vi "Read Best Solution.vi"(8 "error in (no error)":errorcluster, 11 "SA in":refnum<class "SA.lvclass">) -> (0 "error out":errorcluster, 2 "Solution":T1, 3 "SA out":refnum<class "SA.lvclass">)   [LabVIEW 2013, in "SA.lvclass"]
uses:
  SA.lvclass
  Controls/Solution_SA.ctl
  SA.lvclass/SA.ctl
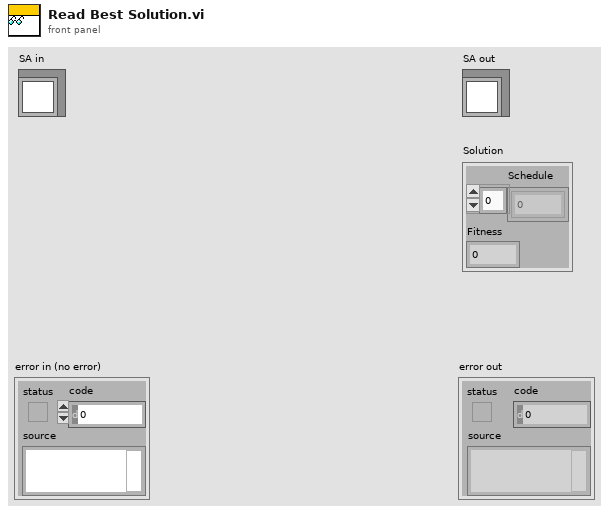
[diagram p1: front panel]
types:
  T1 = typedef "Solution_SA.ctl" = cluster{"Schedule":u16[], "Fitness":i16}
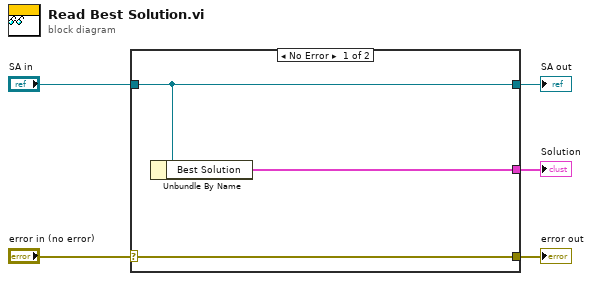
[diagram p0: block diagram]
diagram:
  n1 = case shown="No Error" "error in (no error)" {
    selector: "error in (no error)" -> [w8 w9]
    tunnel: [w8 w9] -> w4
    tunnel: [w7 w10] -> w2
    tunnel: "SA in" -> [w7 w10]
    tunnel: [w6 _] -> w1
    frame No Error {
      n2 = Unbundle By Name(w7) -> ("Best Solution"=w6:T1)
    }
    frame Error {
    }
  }
  "error out" <- w4
  "SA out" <- w2
  "Solution" <- w1
